vi "Table, Set Active Cell Style.vi"(5 "Enable (T)":bool=TRUE, 6 "error in":errorcluster, 7 "Style Default":T1={"BGColor"=16777215, "FontColor"=0, "Italic"=FALSE, "Bold"=FALSE}, 8 "Style Enabled":T1={"BGColor"=16777088, "FontColor"=0, "Italic"=TRUE, "Bold"=TRUE}, 9 "Tbl Refnum":refnum<vi>) -> (0 "error out":errorcluster, 3 "Tbl Refnum out":refnum<vi>)   [LabVIEW 2010]
doc: "Sets the active table cell background color, font color, italic, and bold attributes."
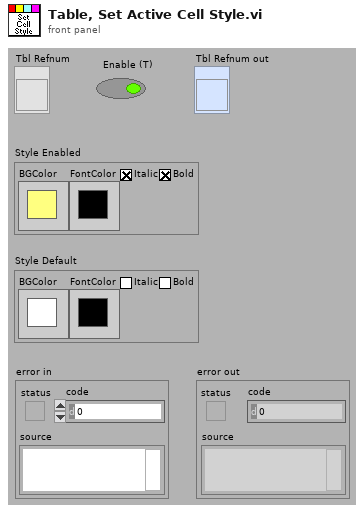
[diagram p1: front panel]
types:
  T1 = cluster{"BGColor":u32, "FontColor":u32, "Italic":bool, "Bold":bool}
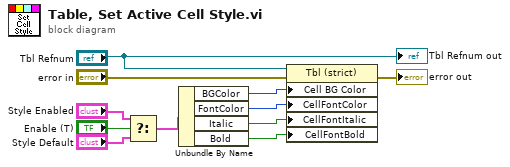
[diagram p0: block diagram]
diagram:
  n1 = Select(t="Style Enabled", s="Enable (T)", f="Style Default") -> (s? t:f=w5:T1)
  n2 = Unbundle By Name(w5) -> ("BGColor"=w4:u32, "FontColor"=w3:u32, "Italic"=w2:bool, "Bold"=w1:bool)
  n3 = property class="Tbl (strict)"(reference="Tbl Refnum", error in="error in", "Cell BG Color"=w4, "CellFontColor"=w3, "CellFontItalic"=w2, "CellFontBold"=w1) -> (error out=→"error out":errorcluster)  [unwired: 1 out]
  "Tbl Refnum out" <- "Tbl Refnum"
